vi "Fnc Global.vi"(3 "error in (no error)":errorcluster, 5 "Command":enum8{"Increment", "Reset", "Get Count"}(ring)) -> (0 "error out":errorcluster, 2 "Numeric":i32)   [LabVIEW 2014]
panel:
  in  "Boolean":bool
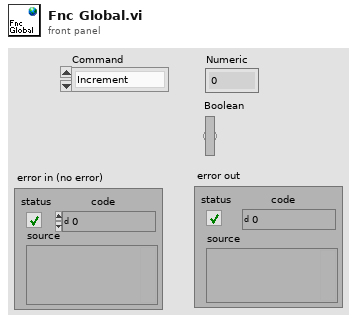
[diagram p1: front panel]
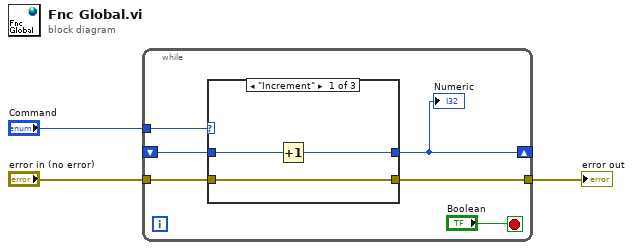
[diagram p0: block diagram]
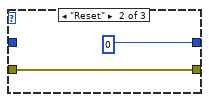
[diagram p2: hidden frame]
diagram:
  n1 = while {
    tunnel: "Command" -> [w9]
    shift-right: [w7] -> _
    shift-left: _ -> [w8]
    tunnel: [w6] -> w3
    tunnel: "error in (no error)" -> [w5]
    stop <- "Boolean" stop-if-true
    n2 = case shown="\"Increment\"" w9 {
      tunnel: w8 -> [w12 _ w16]
      tunnel: [w11 0 w16] -> w7
      tunnel: [w10 w13 w15] -> w6
      tunnel: w5 -> [w10 w13 w15]
      frame "Increment" {
        n3 = Increment(x=w12) -> (x+1=w11:i32)
      }
      frame "Reset" {
      }
      frame "Get Count", Default {
      }
    }
    "Numeric" <- w7
  }
  "error out" <- w3
